vi "Solenoid state setpoint to solenoid channel override.vi"(7 "Solenoid override 1":T2) -> (6 "Open":T1, 10 "Close":T1)   [LabVIEW 2010]
uses:
  Solenoid overide values.ctl
  solenoid channel override.ctl
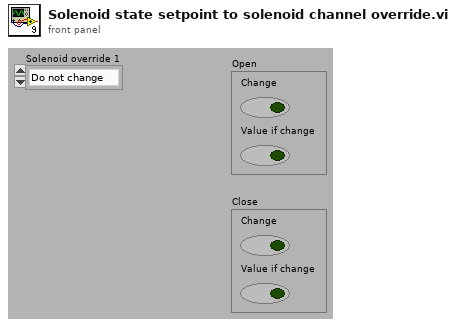
[diagram p1: front panel]
types:
  T1 = typedef "solenoid channel override.ctl" = cluster{"Change":bool, "Value if change":bool}
  T2 = typedef "Solenoid overide values.ctl" = enum16{"Do not change", "Open", "Close", "NA (0-0)", "NA (1-1)"}
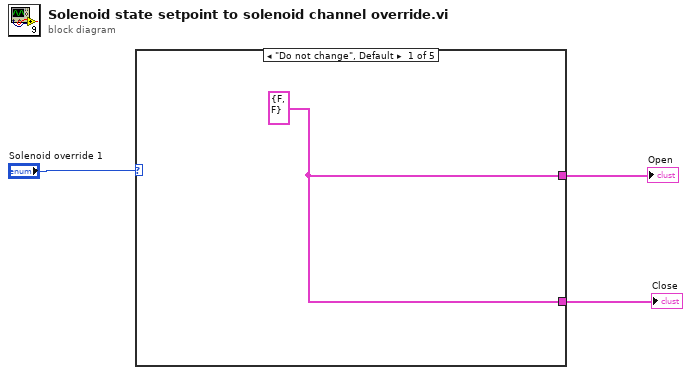
[diagram p0: block diagram]
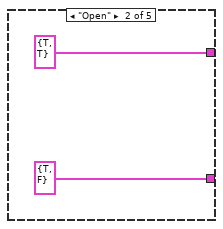
[diagram p2: hidden frame]
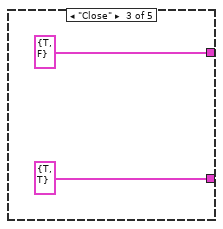
[diagram p3: hidden frame]
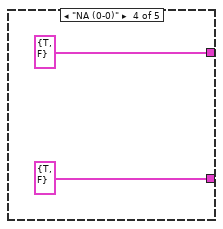
[diagram p4: hidden frame]
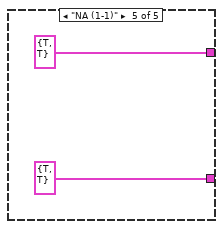
[diagram p5: hidden frame]
diagram:
  n1 = case shown="\"Do not change\", Default" "Solenoid override 1" {
    tunnel: [w4 T1 {"Change"=TRUE, "Value if change"=TRUE} ("Open") T1 {"Change"=TRUE, "Value if change"=FALSE} ("Open") T1 {"Change"=TRUE, "Value if change"=FALSE} ("Open") T1 {"Change"=TRUE, "Value if change"=TRUE} ("Open")] -> w2
    tunnel: [w4 T1 {"Change"=TRUE, "Value if change"=FALSE} ("Open") T1 {"Change"=TRUE, "Value if change"=TRUE} ("Open") T1 {"Change"=TRUE, "Value if change"=FALSE} ("Open") T1 {"Change"=TRUE, "Value if change"=TRUE} ("Open")] -> w1
    frame "Do not change", Default {
      w4 = T1 {"Change"=FALSE, "Value if change"=FALSE} ("Open")
    }
    frame "Open" {
    }
    frame "Close" {
    }
    frame "NA (0-0)" {
    }
    frame "NA (1-1)" {
    }
  }
  "Open" <- w2
  "Close" <- w1
